vi "RefreshEntireTreeWithGlyphManager.vi"(7 "calling VI":refnum<vi>, 8 "error in":errorcluster, 9 "glyph manager":T1, 10 "array":T3[](array[typedef]), 11 "tree ref in":refnum<vi>) -> (0 "error out":errorcluster, 1 "glyph manager out":T1)   [LabVIEW 2025, in "CEF.lvlib"]
doc: "This VI refreshes the complete tree based on the node summary Copyright 2017 National Instruments Corporation\n\nLicensed under the Apache License, Version 2.0 (the \"License\"); you may not use this file except in compliance with the License. You may obtain a copy of the License at http://www.apache.org/licenses/LICENSE-2.0\nUnless required by applicable law or agreed to in writing, software distributed under the License is distributed on an \"AS IS\" BASIS, WITHOUT WARRANTIES OR CONDITIONS OF ANY KIND, either express or implied. See the License for the specific language governing permissions and limitations under the License."
uses:
  CEF.lvlib
  Node/Summary.ctl
  glyph manager/glyph manager.ctl
  <vilib>/picture/picture.llb/imagedata.ctl
  Node/CEF_Node.lvclass
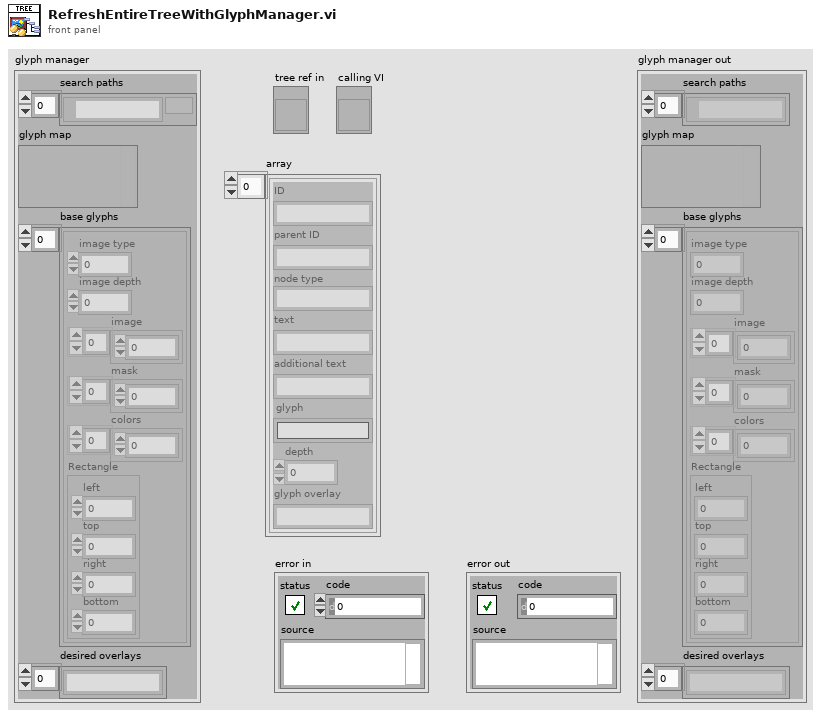
[diagram p1: front panel]
types:
  T1 = typedef "CEF.lvlib/glyph manager.ctl" = cluster{"search paths":path[], "glyph map":variant, "base glyphs":T2[], "desired overlays":string[]}
  T2 = typedef "imagedata.ctl" = cluster{"image type":i32, "image depth":i32, "image":u8[], "mask":u8[], "colors":u32[], "Rectangle":cluster{"left":i16, "top":i16, "right":i16, "bottom":i16}}
  T3 = typedef "CEF.lvlib/CEF_Node.lvclass/Summary.ctl" = cluster{"ID":string, "parent ID":string, "node type":string, "text":string, "additional text":string, "glyph":string, "depth":i32, "glyph overlay":string}
  T4 = cluster{"Left Cell String":string, "Child text":string[], "Child Tag":string, "Item Indent":i32, "Child Only?":bool, "glyph Index":i32}
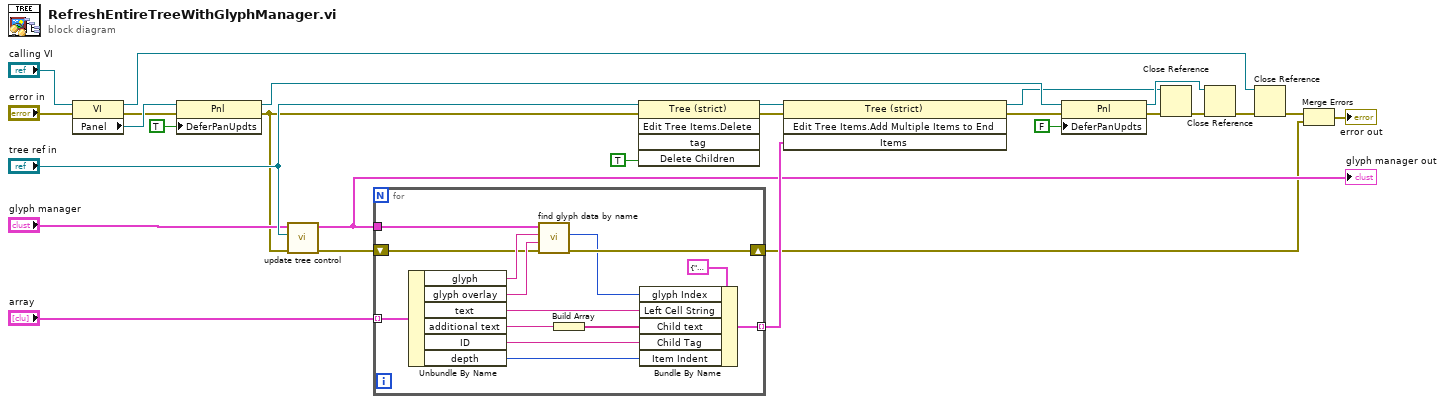
[diagram p0: block diagram]
diagram:
  n1 = property class="VI"(reference="calling VI", error in="error in") -> (reference out=w19:refnum<vi>, error out=w4:errorcluster, "Panel"=w26:refnum<vi>)
  n2 = property class="Pnl"(reference=w26, error in=w4, "DeferPanUpdts"=TRUE ("Defer Panel Updates")) -> (reference out=w23:refnum<vi>, error out=w2:errorcluster)
  n3 = call "update tree control.vi"("error in"=w2, "tree reference"="tree ref in", "glyph manager in"="glyph manager") -> ("error out"=w1:errorcluster, "glyph manager out"=w6:T1)  [unwired: 7 in]
  "glyph manager out" <- w6
  n4 = for {
    tunnel: "array" -> [w41] mode=indexing
    tunnel: [w39] -> w13 mode=indexing
    tunnel: w6 -> [w32]
    shift-right: [w33] -> w3
    shift-left: w1 -> [w28]
    n5 = Unbundle By Name(w41) -> ("glyph"=w31:string, "glyph overlay"=w30:string, "text"=w38:string, "additional text"=w36:string, "ID"=w35:string, "depth"=w34:i32)
    n6 = call "find glyph data by name.vi"("error in"=w28, "overlay"=w30, "name"=w31, "glyph manager in"=w32) -> ("error out"=w33:errorcluster, "symbol index"=w29:i32)  [unwired: 4 in, 2 out]
    n7 = Build Array(w36) -> (w37:string[])
    n8 = Bundle By Name(cluster=T4 {"Left Cell String"="", "Child text"=[], "Child Tag"="", "Item Indent"=0, "Child Only?"=FALSE, "glyph Index"=0} ("Item"), "glyph Index"=w29, "Left Cell String"=w38, "Child text"=w37, "Child Tag"=w35, "Item Indent"=w34) -> (w39:T4)
  }
  n9 = invoke class="Tree (strict)" method="Edit Tree Items.Delete"(reference="tree ref in", error in=w2, "Delete Children"=TRUE ("Delete Children?")) -> (reference out=w15:refnum<vi>, error out=w12:errorcluster)  [unwired: 2 in, 3 out]
  n10 = invoke class="Tree (strict)" method="Edit Tree Items.Add Multiple Items to End"(reference=w15, error in=w12, "Items"=w13) -> (reference out=w14:refnum<vi>, error out=w11:errorcluster)  [unwired: 1 in, 2 out]
  n11 = property class="Pnl"(reference=w23, error in=w11, "DeferPanUpdts"=FALSE ("Defer Panel Updates")) -> (reference out=w20:refnum<vi>, error out=w22:errorcluster)
  n12 = Close Reference(reference=w14, error in (no error)=w22) -> (error out=w21:errorcluster)
  n13 = Close Reference(reference=w20, error in (no error)=w21) -> (error out=w18:errorcluster)
  n14 = Close Reference(reference=w19, error in (no error)=w18) -> (error out=w9:errorcluster)
  n15 = Merge Errors(w9, w3) -> (→"error out":errorcluster)
